vi "LSCI332 SetCtrlMode.vi"(0 "VISA Rsrc":refnum<visa-resource-name>="GPIB0::12::INSTR", 5 "Boucle(1)":u32(ring) caption="Boucle" items=["Boucle 1", "Boucle 2"], 7 "Mode":u32(ring)=1 items=["Manual PID"=1, "Zone"=2, "Open Loop"=3, "AutoTune PID"=4, "AutoTune PI"=5, "AutoTune P"=6], 11 "error in (no error)":errorcluster) -> (15 "error out":errorcluster)   [LabVIEW 2012]
doc: "Ce VI écrit les paramètres limites de contrôle dans le contrôleur."
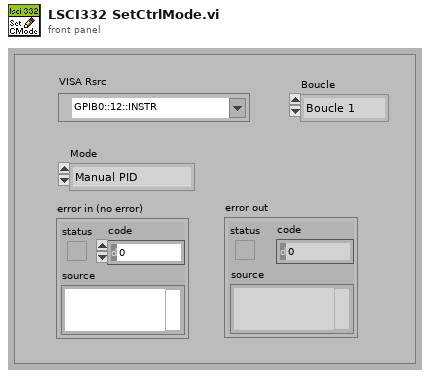
[diagram p1: front panel]
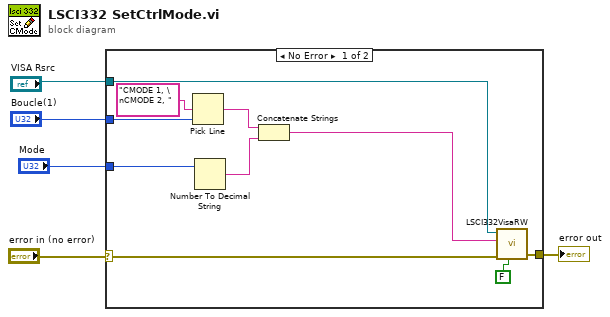
[diagram p0: block diagram]
diagram:
  n1 = case shown="No Error" "error in (no error)" {
    selector: "error in (no error)" -> [w13 w16]
    tunnel: "VISA Rsrc" -> [w15 _]
    tunnel: "Boucle(1)" -> [w10 _]
    tunnel: [w14 w16] -> w3
    tunnel: "Mode" -> [w9 _]
    frame No Error {
      n2 = Pick Line(multi-line string="CMODE 1, \nCMODE 2, ", line index=w10) -> (output string=w8:string)  [unwired: 1 in]
      n3 = Number To Decimal String(number=w9) -> (decimal integer string=w7:string)  [unwired: 1 in]
      n4 = Concatenate Strings(w8, w7) -> (w6:string)
      n5 = call <userlib>:"LSCI332VisaRW.vi"("Lecture?(T)"=FALSE, "error in (no error)"=w13, "ChaineCom"=w6, "VISA Rsrc"=w15) -> ("error out"=w14:errorcluster)  [unwired: 3 in, 3 out]
    }
    frame Error {
    }
  }
  "error out" <- w3
